vi "Update Room Details.vi"(0 "Guest Manager Model in":refnum<class "Guest Manager Model.lvclass">, 5 "Guest Contact Number Out":string caption="Guest Contact Number", 7 "Primary Guest Name Out":string caption="Primary Guest Name", 9 "Bill Summary":string, 11 "error in (no error)":errorcluster) -> (4 "Guest Manager Model out":refnum<class "Guest Manager Model.lvclass">, 15 "error out":errorcluster)   [LabVIEW 2023, in "Guest Manager Model.lvlib" / "Guest Manager Model.lvclass"]
uses:
  Guest Manager Model.lvclass
  <vilib>/ActorFramework/Actor/Actor.lvclass/Actor.ctl
  <vilib>/ActorFramework/Message Enqueuer/Message Enqueuer.lvclass/Message Enqueuer.ctl
  Guest Manager UI/Guest Manager UI Messages/Update Room Details Msg/Update Room Details Msg.lvclass/Update Room Details Msg.ctl
  <vilib>/ActorFramework/Message Enqueuer/Init from Existing Queue.vi
  <vilib>/ActorFramework/Message Enqueuer/Enqueue.vi
  Guest Manager UI/Guest Manager UI Messages/Update Room Details Msg/Update Room Details Msg.lvclass
  <vilib>/ActorFramework/Message Priority Queue/Priority Enqueue.vi
  <vilib>/ActorFramework/Message Enqueuer/Message Enqueuer.lvclass
  Guest Manager Model.lvclass/Guest Manager Model.ctl
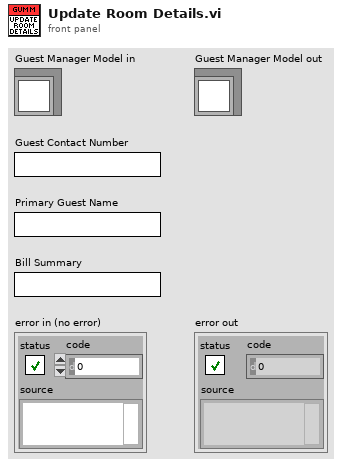
[diagram p1: front panel]
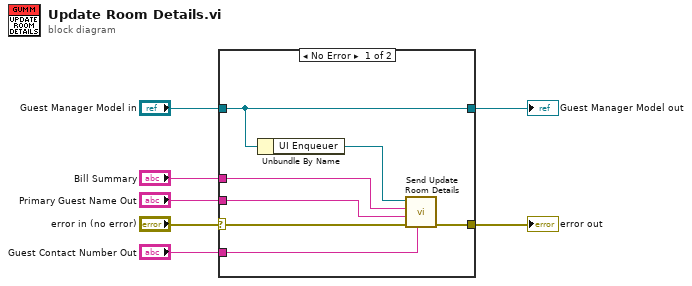
[diagram p0: block diagram]
diagram:
  n1 = case shown="No Error" "error in (no error)" {
    selector: "error in (no error)" -> [w14 w16]
    tunnel: [w13 w16] -> w6
    tunnel: [w9 w15] -> w4
    tunnel: "Guest Manager Model in" -> [w9 w15]
    tunnel: "Bill Summary" -> [w11 _]
    tunnel: "Guest Contact Number Out" -> [w12 _]
    tunnel: "Primary Guest Name Out" -> [w10 _]
    frame No Error {
      n2 = Unbundle By Name(w9) -> ("UI Enqueuer"=w8:refnum<class "Message Enqueuer.lvclass">)
      n3 = call "Send Update Room Details.vi"("Guest Contact Number Out"=w12, "error in (no error)"=w14, "Primary Guest Name Out"=w10, "Bill Summary"=w11, "Message Enqueuer"=w8) -> ("error out"=w13:errorcluster)  [unwired: 5 in, 1 out]
    }
    frame Error {
    }
  }
  "error out" <- w6
  "Guest Manager Model out" <- w4
